vi "BoilerRoom AlarmGraph 2.vi"() -> ()   [LabVIEW 2023]
uses:
  <vilib>/Utility/error.llb/Trim Whitespace One-Sided.vi
  Heater.vi
  AC.vi
panel:
  out "Message 2":string
  out "Waveform Chart 2":dbl[][](graph)
  out "Waveform Chart":i32(graph)
  out "Message":string
  out "Alarm":bool
  out "temp":dbl
  in  "?":dbl(knob) min=0.0 max=2.0 step=1.0 scale=0.0..2.0
  in  "stop":bool
  out "Thermometer":dbl(slide) scale=0.0..100.0
  in  "min temp":dbl=20.0
  in  "max temp":dbl=80.0
  in  "Automatic / Manual":bool
  out "AC":bool
  out "Heater":bool
  # "Heater"
  # "OFF"
  # "AC"
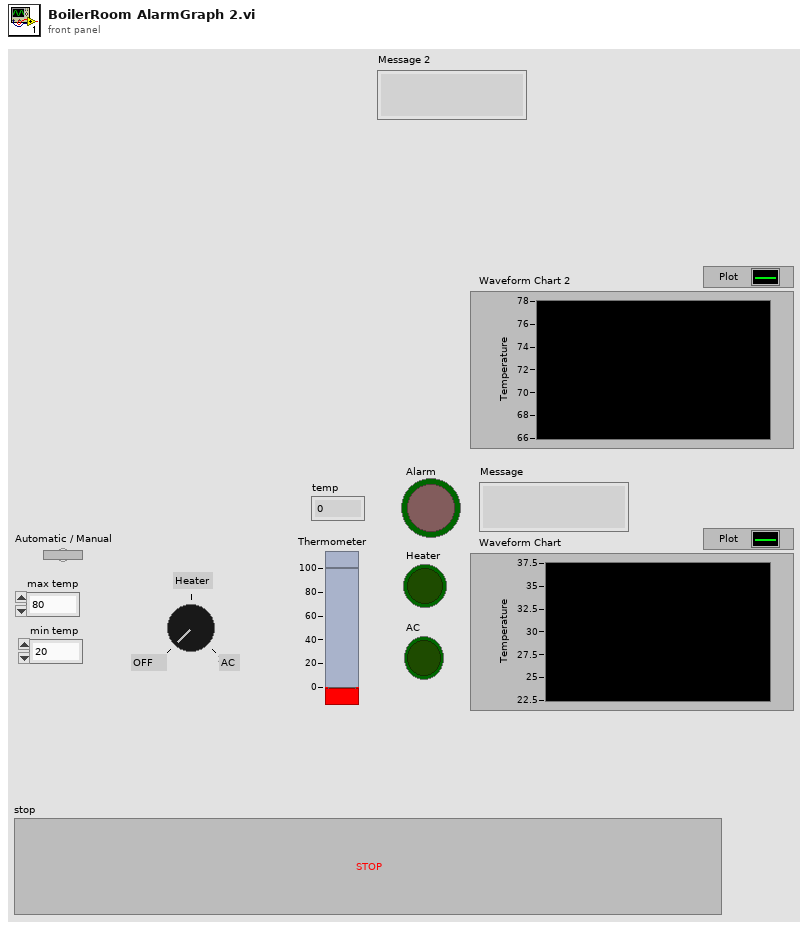
[diagram p1: front panel]
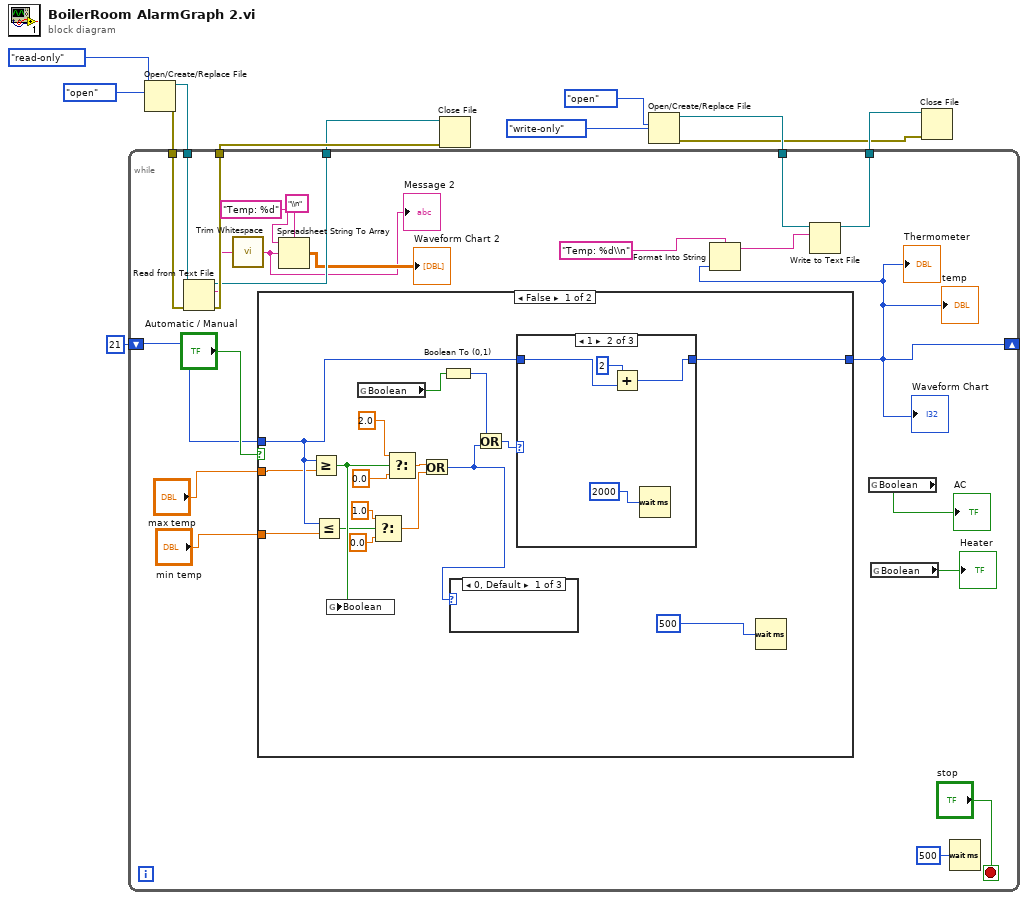
[diagram p0: block diagram]
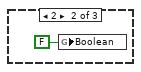
[diagram p2: hidden frame]
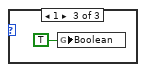
[diagram p3: hidden frame]
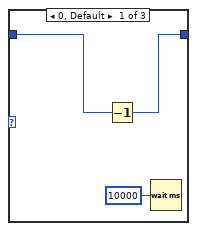
[diagram p4: hidden frame]
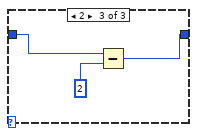
[diagram p5: hidden frame]
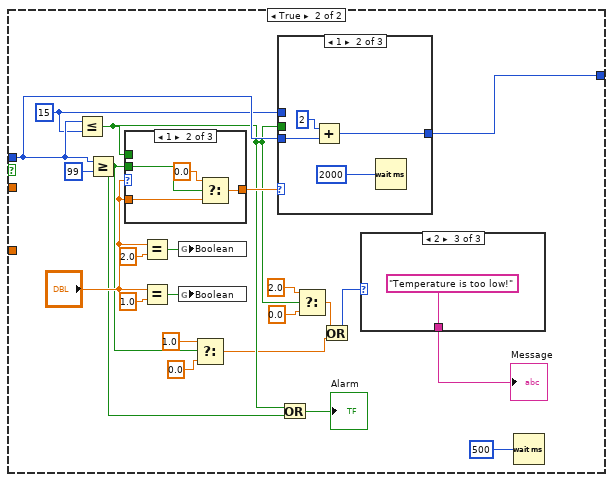
[diagram p6: hidden frame]
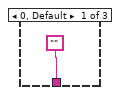
[diagram p7: hidden frame]
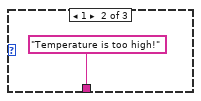
[diagram p8: hidden frame]
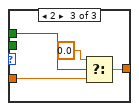
[diagram p10: hidden frame]
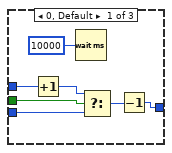
[diagram p11: hidden frame]
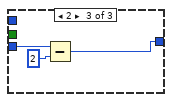
[diagram p12: hidden frame]
diagram:
  n1 = Open/Create/Replace File(operation (0:open)=enum16{"open", "replace"}."open", access (0:read/write)=enum16{"read/write", "read-only", "write-only"}."read-only") -> (refnum out=w3:refnum<file>, error out=w4:errorcluster)  [unwired: 4 in, 1 out]
  n2 = Open/Create/Replace File(operation (0:open)=enum16{"open", "replace"}."open", access (0:read/write)=enum16{"read/write", "read-only", "write-only"}."write-only") -> (refnum out=w8:refnum<file>, error out=w7:errorcluster)  [unwired: 4 in, 1 out]
  n3 = while {
    shift-right: [w23] -> _
    shift-left: 21 -> [w27]
    tunnel: w8 -> [w26]
    tunnel: [w25] -> w10
    tunnel: w4 -> [w21]
    tunnel: w3 -> [w20]
    tunnel: [w19] -> w2
    tunnel: [w18] -> w1
    stop <- "stop" stop-if-true
    n4 = Read from Text File(file (use dialog)=w20, error in=w21) -> (refnum out=w18:refnum<file>, text=w17:string, error out=w19:errorcluster)  [unwired: 2 in, 1 out]
    n5 = call <vilib>:"Trim Whitespace.vi"("string"=w17) -> ("trimmed string"=w13:string)  [unwired: 1 in]
    "Message 2" <- w13
    n6 = case shown="False" "Automatic / Manual" {
      tunnel: w27 -> [w44 w78]
      tunnel: "max temp" -> [w43 _]
      tunnel: "min temp" -> [w42 _]
      tunnel: [w46 w84] -> w23
      frame False {
        n7 = Greater Or Equal?(x=w44, y=w43) -> (x >= y?=w40:bool)
        n8 = Less Or Equal?(x=w44, y=w42) -> (x <= y?=w39:bool)
        n9 = global write "AC.vi" "Boolean"(w40) -> ()
        n10 = global read "Heater.vi" "Boolean"() -> (w35:bool)
        n11 = Select(t=1.0, s=w39, f=0.0) -> (s? t:f=w41:dbl)
        n12 = Select(t=2.0, s=w40, f=0.0) -> (s? t:f=w47:dbl)
        n13 = Or(x=w47, y=w41) -> (x .or. y?=w38:i32)
        n14 = Boolean To (0,1)(Boolean=w35) -> (0, 1=w36:i16)
        n15 = case shown="0, Default" w38 {
          frame 0, Default {
          }
          frame 2 {
            n16 = global write "Heater.vi" "Boolean"(FALSE ("Boolean")) -> ()
          }
          frame 1 {
            n17 = global write "Heater.vi" "Boolean"(TRUE ("Boolean")) -> ()
          }
        }
        n18 = Or(x=w36, y=w38) -> (x .or. y?=w37:i32)
        n19 = case shown="1" w37 {
          tunnel: w44 -> [w56 w60 w63]
          tunnel: [w55 w58 w62] -> w46
          frame 0, Default {
            n20 = Decrement(x=w56) -> (x-1=w55:i32)
            n21 = Wait (ms)(milliseconds to wait=u32 10000) -> ()  [unwired: 1 out]
          }
          frame 1 {
            n22 = Add(x=2, y=w60) -> (x+y=w58:i32)
            n23 = Wait (ms)(milliseconds to wait=u32 2000) -> ()  [unwired: 1 out]
          }
          frame 2 {
            n24 = Subtract(x=w63, y=2) -> (x-y=w62:i32)
          }
        }
        n25 = Wait (ms)(milliseconds to wait=u32 500) -> ()  [unwired: 1 out]
      }
      frame True {
        w75 = 15
        n26 = Less Or Equal?(x=w78, y=w75) -> (x <= y?=w70:bool)
        n27 = Greater Or Equal?(x=w78, y=99 ("x")) -> (x >= y?=w69:bool)
        n28 = case shown="1" "?" {
          tunnel: "?" -> [w89 w90 w95]
          tunnel: [w89 w92 w96] -> w83
          tunnel: w69 -> [_ w93 _]
          tunnel: w70 -> [_ _ w97]
          frame 0, Default {
          }
          frame 1 {
            n29 = Select(t=0.0 ("f"), s=w93, f=w90) -> (s? t:f=w92:dbl)
          }
          frame 2 {
            n30 = Select(t=0.0, s=w97, f=w95) -> (s? t:f=w96:dbl)
          }
        }
        n31 = Equal?(x="?", y=2.0) -> (x = y?=w79:bool)
        n32 = Equal?(x="?", y=1.0) -> (x = y?=w81:bool)
        n33 = global write "AC.vi" "Boolean"(w79) -> ()
        n34 = global write "Heater.vi" "Boolean"(w81) -> ()
        n35 = Select(t=1.0, s=w69, f=0.0) -> (s? t:f=w66:dbl)
        n36 = case shown="1" w83 {
          tunnel: w78 -> [w101 w108 w111]
          tunnel: [w104 w107 w110] -> w84
          tunnel: w70 -> [w102 _ _]
          tunnel: w75 -> [w99 _ _]
          frame 0, Default {
            n37 = Increment(x=w99) -> (x+1=w98:i32)
            n38 = Wait (ms)(milliseconds to wait=u32 10000) -> ()  [unwired: 1 out]
            n39 = Select(t=w98, s=w102, f=w101) -> (s? t:f=w100:i32)
            n40 = Decrement(x=w100) -> (x-1=w104:i32)
          }
          frame 1 {
            n41 = Add(x=2, y=w108) -> (x+y=w107:i32)
            n42 = Wait (ms)(milliseconds to wait=u32 2000) -> ()  [unwired: 1 out]
          }
          frame 2 {
            n43 = Subtract(x=w111, y=2) -> (x-y=w110:i32)
          }
        }
        n44 = Or(x=w70, y=w69) -> (x .or. y?=→"Alarm":bool)
        n45 = Select(t=2.0, s=w70, f=0.0) -> (s? t:f=w65:dbl)
        n46 = Or(x=w65, y=w66) -> (x .or. y?=w64:i32)
        n47 = case shown="2" w64 {
          tunnel: ["" "Temperature is too high!" "Temperature is too low!"] -> w68
          frame 0, Default {
          }
          frame 1 {
          }
          frame 2 {
          }
        }
        "Message" <- w68
        n48 = Wait (ms)(milliseconds to wait=u32 500) -> ()  [unwired: 1 out]
      }
    }
    "Thermometer" <- w23
    "temp" <- w23
    "Waveform Chart" <- w23
    n49 = Spreadsheet String To Array(delimiter (Tab)="\\n", format string="Temp: %d", spreadsheet string=w13) -> (array=→"Waveform Chart 2":dbl[][])  [unwired: 1 in]
    n50 = Format Into String(format string="Temp: %d\\n", w23) -> (resulting string=w22:string)  [unwired: 2 in, 1 out]
    n51 = Write to Text File(file (use dialog)=w26, text=w22) -> (refnum out=w25:refnum<file>)  [unwired: 2 in, 2 out]
    n52 = global read "AC.vi" "Boolean"() -> (→"AC":bool)
    n53 = global read "Heater.vi" "Boolean"() -> (→"Heater":bool)
    n54 = Wait (ms)(milliseconds to wait=u32 500) -> ()  [unwired: 1 out]
  }
  n55 = Close File(refnum=w1, error in=w2) -> ()  [unwired: 2 out]
  n56 = Close File(refnum=w10, error in=w7) -> ()  [unwired: 2 out]
